vi "Write Return Address.vi"(9 "Return Priority (Normal)":T1=enum."Normal", 10 "Return Enqueuer":refnum<class "Message Enqueuer.lvclass">, 11 "RoundTripMessage In":refnum<class "RoundTripMessage.lvclass">) -> (3 "RoundTripMessage Out":refnum<class "RoundTripMessage.lvclass">)   [LabVIEW 2020, in "RoundTripMessage.lvclass"]
doc: "<License>\nCopyright © 2017 Composed Systems, LLC | All rights reserved\nwww.composed.io\n\nAuthor: Ethan Stern <ethan.stern@composed.io>\n\nThis software is provided \"AS IS\" WITHOUT WARRANTIES, either express or implied, AND IS FOR EDUCATIONAL PURPOSES ONLY.\n</License>"
uses:
  <vilib>/gpm_packages/@cs/actor-framework-messages/Source/RoundTripMessage/RoundTripMessage.lvclass
  <vilib>/ActorFramework/Message Enqueuer/Message Enqueuer.lvclass
  <vilib>/ActorFramework/Message Enqueuer/Message Priority.ctl
  <vilib>/gpm_packages/@cs/actor-framework-messages/Source/RoundTripMessage/RoundTripMessage.lvclass/RoundTripMessage.ctl
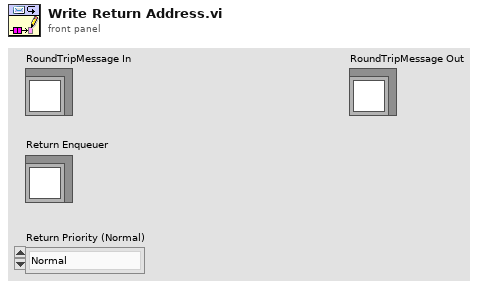
[diagram p1: front panel]
types:
  T1 = typedef "Actor Framework.lvlib/Message Enqueuer.lvclass/Message Priority.ctl" = enum16{"Low", "Normal", "High"}
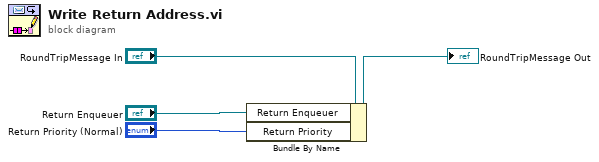
[diagram p0: block diagram]
diagram:
  n1 = Bundle By Name(cluster="RoundTripMessage In", "Return Enqueuer"="Return Enqueuer", "Return Priority"="Return Priority (Normal)") -> (→"RoundTripMessage Out":refnum<class "RoundTripMessage.lvclass">)
